vi "save method.vi"(7 "SD method":T1 {"method array"."offset" format="%.2f"; "method array"."amplitude" format="%.2f"; "method array"."cycles/repeat period" min=1}) -> ()   [LabVIEW 2010]
uses:
  file action.ctl
  SDMethod.ctl
panel:
  # "ticks"
  # "hz"
  # "ticks"
  # "ticks"
  # "volts"
  # "volts"
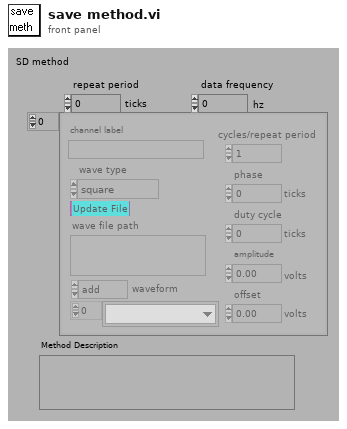
[diagram p1: front panel]
types:
  T1 = typedef "SDMethod.ctl" = cluster{"method array":cluster{"wave type":enum16{"off", "square", "sine", "triangle", "sawtooth", "from file", "wavemaker", "flume pump"}, "cycles/repeat period":u32, "phase":i32, "duty cycle":u32, "wave file path":path, "amplitude":dbl, "channel label":string, "Update":bool, "offset":dbl, " waveform":u16[], "Function":enum16{"add", "multiply"}}[], "Method Description":string, "data frequency":u32, "repeat period":u32}
  T2 = typedef "file action.ctl" = enum16{"Save", "Open"}
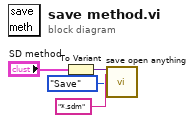
[diagram p0: block diagram]
diagram:
  n1 = To Variant(anything="SD method") -> (Variant=w3:variant)
  n2 = call "save open anything.vi"("Variant"=w3, "Action"=file_action."Save", "pattern"="*.sdm") -> ()  [unwired: 4 in, 4 out]
